vi "Hypergeometric PF.vi"(8 "n":i32=20, 9 "k":i32=30, 10 "M":i32=100, 11 "x":i32=1) -> (0 "error":i32, 3 "prob(x)":dbl=0.003553328058550957)   [LabVIEW 2020, in "NI_Gmath.lvlib"]
doc: "Computes the discrete probability function (PF), or the probability that the random variate X, where X describes the selected distribution type, takes on the value <B>n</B>. You must manually select the polymorphic instance to use."
uses:
  <vilib>/gmath/NI_Gmath.lvlib
panel:
  # "Hypergeometric PF"
  # "size of population"
  # "items"
  # "samples drawn"
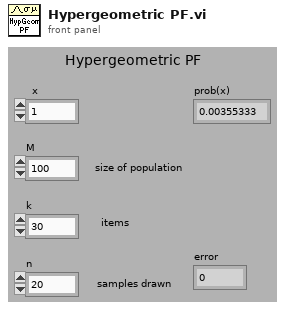
[diagram p1: front panel]
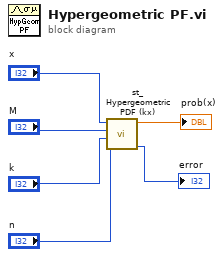
[diagram p0: block diagram]
diagram:
  n1 = call <vilib>:"st_Hypergeometric PDF (kx).vi"("n = samples drawn"="n", "k = items"="k", "M = size of population"="M", "x"="x") -> ("error"=→"error":i32, "pdf(x)"=→"prob(x)":dbl)  [unwired: 6 in]
